vi "ScaleRawData.vi"(4 "Vx,Vy,Vsum as signals or\ntrue X,Y,Z signal (1,default)":bool=TRUE, 5 "error in (no error)":errorcluster, 6 "All DAQ channels":T3, 7 "Scale Option":i32(ring)=2 items=["ScaleButDoNotCalculatePsi", "CalculatePsi, ButDoNotCompensate", "CompensationAllSignalsByCalcuatedPsi", "DoNotScale(ReadRawVoltageSignals)"], 8 "Params in":T8={"TaskIDs"={"DAQ tasks"={"Px taskID"=0, "Py taskID"=0, "Pz taskID"=0, "AOM taskID"=0, "Clock taskID"=0, "AI taskID"=0}, "DVEHandle"=refnum}, "Manual Control"={"Rotation Control"={"Phase"=0.0, "A amp (0-120)"=75.0, "B amp (0-120)"=53.3, "mean freq  [MHz]\ndefault 39.99"=40.0, "freq difference [Hz]"=2.0, "Enable A"=TRUE, "Enable B"=TRUE}, "X piezo\n [nm]"=0.0, "Y peizo\n [nm]"=0.0, "trap height\n [nm]"=5.012658227848101, "AOM0 \nPower"=0.2}, "Piezo Calibr"={"Px2Vx(AO)"=nan, "Py2Vy(AO)"=nan, "Pz2Vz(AO)"=nan, "Min Px"=nan, "Min Py"=nan, "Min Pz"=nan, "Max Px"=nan, "Max Py"=nan, "Max Pz"=nan, "Vx0 (V)"=nan, "Vy0 (V)"=nan, "Vz0 (V)"=nan}, "Instrument Calibr"={"Angular compensation coeffs"=[], "TetherCenter"={"TrapX_AO 0 [nm]"=nan, "TrapY_AO 0 [nm]"=nan, "TrapZ_AO 0 [nm]"=nan}, "XYZsignal baseline"={"Xsignal0"=nan, "Ysignal0"=nan, "Zsignal0"=nan, "Zsig slope"=nan, "Z bead0"=nan}, "S and P to Vs0"={"Vs0/P"=1.0, "Vs0/S"=1.0}, "Psi"=0.0, "ePS:eRL drift correlation"={"Interc P"=nan, "Slope P"=nan, "Interc S"=nan, "Slope S"=nan}, "Current piezo volt AO"={"Vpx_AO [V]"=nan, "Vpy_AO [V]"=nan, "Vpz_AO [V]"=nan}}, "Cylinder Calibr"={"ZStiff"=nan, "Zsens"=nan, "AngStiff"=nan, "XStiff"=nan, "Xsens"=nan, "MaxEllip"=nan, "YStiff"=nan, "Ysens"=nan, "FocalShift"=nan, "Sfz"=nan, "1/Sz"=nan, "Stau"=nan, "Sfx"=nan, "1/Sx"=nan, "1/Sang"=nan, "Sfy"=nan, "1/Sy"=nan, "1/focal"=nan, "ZsignalHeightDependence (1/nm)"=0.0}, "DAQParams"={"Buffer size"=nan, "Scanning rate"=nan, "Average"=nan, "Sampling rate"=nan, "set dt"=nan}, "DAQ channel offsets"={"A0 [V]"=0.0, "D0 [V]"=0.0, "P0  [V]"=0.0, "S0 [V]"=0.0, "L0 [V]"=0.0, "R0 [V]"=0.0, "Vpx0 [V]"=0.0, "Vpy0 [V]"=0.0, "Vpz0 [V]"=0.0, "Vsum0 [V]"=0.0, "Vpx_AO0 [V]"=0.0, "Vpy_AO0 [V]"=0.0, "Vpz_AO0 [V]"=0.0}, "Z bead polynomial coeffs"=[nan, nan, nan, nan], "Skip button ref"=refnum, "z bead lookup table"={"z signal"=[], "z bead"=[]}, "SP->power Matrix"=[], "Ms2p"=[], "Mp2s"=[], "Polynomial coeff V_px,y,z 2 position (nm)"=[]} {"Cylinder Calibr"."ZsignalHeightDependence (1/nm)" format="%.4e"; "Instrument Calibr"."Psi" format="%#_2f"; "Manual Control"."Y peizo\n [nm]" step=100.0 scale=0.0..30000.0; "Manual Control"."AOM0 \nPower" scale=0.0..1.0; "Manual Control"."X piezo\n [nm]" step=100.0 scale=0.0..30000.0; "Manual Control"."Rotation Control"."mean freq  [MHz]\ndefault 39.99" min=0.0 step=0.01; "Manual Control"."Rotation Control"."B amp (0-120)" min=0.0 max=120.0 step=0.1 format="%.1f"; "Manual Control"."Rotation Control"."A amp (0-120)" min=0.0 max=120.0 step=0.1 format="%.1f"; "Manual Control"."Rotation Control"."Phase" scale=0.0..360.0; "Manual Control"."trap height\n [nm]" scale=1000.0..7500.0; "TaskIDs"."DAQ tasks"."Px taskID" format="%x"; "TaskIDs"."DAQ tasks"."Py taskID" format="%x"; "TaskIDs"."DAQ tasks"."Pz taskID" format="%x"; "TaskIDs"."DAQ tasks"."AOM taskID" format="%x"; "TaskIDs"."DAQ tasks"."Clock taskID" format="%x"; "TaskIDs"."DAQ tasks"."AI taskID" format="%x"}) -> (0 "error out":errorcluster, 1 "Scaled data":T7, 2 "All DAQ channels out":T3, 3 "Params out":T8={"TaskIDs"={"DAQ tasks"={"Px taskID"=0, "Py taskID"=0, "Pz taskID"=0, "AOM taskID"=0, "Clock taskID"=0, "AI taskID"=0}, "DVEHandle"=refnum}, "Manual Control"={"Rotation Control"={"Phase"=0.0, "A amp (0-120)"=75.0, "B amp (0-120)"=53.3, "mean freq  [MHz]\ndefault 39.99"=40.0, "freq difference [Hz]"=2.0, "Enable A"=TRUE, "Enable B"=TRUE}, "X piezo\n [nm]"=0.0, "Y peizo\n [nm]"=0.0, "trap height\n [nm]"=5.012658227848101, "AOM0 \nPower"=0.2}, "Piezo Calibr"={"Px2Vx(AO)"=nan, "Py2Vy(AO)"=nan, "Pz2Vz(AO)"=nan, "Min Px"=nan, "Min Py"=nan, "Min Pz"=nan, "Max Px"=nan, "Max Py"=nan, "Max Pz"=nan, "Vx0 (V)"=nan, "Vy0 (V)"=nan, "Vz0 (V)"=nan}, "Instrument Calibr"={"Angular compensation coeffs"=[], "TetherCenter"={"TrapX_AO 0 [nm]"=nan, "TrapY_AO 0 [nm]"=nan, "TrapZ_AO 0 [nm]"=nan}, "XYZsignal baseline"={"Xsignal0"=nan, "Ysignal0"=nan, "Zsignal0"=nan, "Zsig slope"=nan, "Z bead0"=nan}, "S and P to Vs0"={"Vs0/P"=1.0, "Vs0/S"=1.0}, "Psi"=0.0, "ePS:eRL drift correlation"={"Interc P"=nan, "Slope P"=nan, "Interc S"=nan, "Slope S"=nan}, "Current piezo volt AO"={"Vpx_AO [V]"=nan, "Vpy_AO [V]"=nan, "Vpz_AO [V]"=nan}}, "Cylinder Calibr"={"ZStiff"=nan, "Zsens"=nan, "AngStiff"=nan, "XStiff"=nan, "Xsens"=nan, "MaxEllip"=nan, "YStiff"=nan, "Ysens"=nan, "FocalShift"=nan, "Sfz"=nan, "1/Sz"=nan, "Stau"=nan, "Sfx"=nan, "1/Sx"=nan, "1/Sang"=nan, "Sfy"=nan, "1/Sy"=nan, "1/focal"=nan, "ZsignalHeightDependence (1/nm)"=0.0}, "DAQParams"={"Buffer size"=nan, "Scanning rate"=nan, "Average"=nan, "Sampling rate"=nan, "set dt"=nan}, "DAQ channel offsets"={"A0 [V]"=0.0, "D0 [V]"=0.0, "P0  [V]"=0.0, "S0 [V]"=0.0, "L0 [V]"=0.0, "R0 [V]"=0.0, "Vpx0 [V]"=0.0, "Vpy0 [V]"=0.0, "Vpz0 [V]"=0.0, "Vsum0 [V]"=0.0, "Vpx_AO0 [V]"=0.0, "Vpy_AO0 [V]"=0.0, "Vpz_AO0 [V]"=0.0}, "Z bead polynomial coeffs"=[nan, nan, nan, nan], "Skip button ref"=refnum, "z bead lookup table"={"z signal"=[], "z bead"=[]}, "SP->power Matrix"=[], "Ms2p"=[], "Mp2s"=[], "Polynomial coeff V_px,y,z 2 position (nm)"=[]} {"Cylinder Calibr"."ZsignalHeightDependence (1/nm)" format="%.4e"; "Instrument Calibr"."Psi" format="%#_2f"; "Manual Control"."Y peizo\n [nm]" step=100.0 scale=0.0..30000.0; "Manual Control"."AOM0 \nPower" scale=0.0..1.0; "Manual Control"."X piezo\n [nm]" step=100.0 scale=0.0..30000.0; "Manual Control"."Rotation Control"."mean freq  [MHz]\ndefault 39.99" min=0.0 step=0.01; "Manual Control"."Rotation Control"."B amp (0-120)" min=0.0 max=120.0 step=0.1 format="%.1f"; "Manual Control"."Rotation Control"."A amp (0-120)" min=0.0 max=120.0 step=0.1 format="%.1f"; "Manual Control"."Rotation Control"."Phase" scale=0.0..360.0; "Manual Control"."trap height\n [nm]" scale=1000.0..7500.0; "TaskIDs"."DAQ tasks"."Px taskID" format="%x"; "TaskIDs"."DAQ tasks"."Py taskID" format="%x"; "TaskIDs"."DAQ tasks"."Pz taskID" format="%x"; "TaskIDs"."DAQ tasks"."AOM taskID" format="%x"; "TaskIDs"."DAQ tasks"."Clock taskID" format="%x"; "TaskIDs"."DAQ tasks"."AI taskID" format="%x"})   [LabVIEW 2020, in "SignalConverson.lvlib"]
uses:
  SignalConverson.lvlib
  Initialization/Param.ctl
  Initialization/ManualCtrl.ctl
  Initialization/DVESetting.ctl
  Initialization/CylinderCalibrNew.ctl
  DAQChannelOffsets.ctl
  <vilib>/Analysis/Matrix/Datatypes/RealMatrix.ctl
  DAQChannelRawData.ctl
  ScaledData.ctl
  Measrured TrapXYZ.ctl
  Data Before Angle Compensation.ctl
  Angle compensated data.ctl
  XYZ Signals.ctl
  Set TrapXYZ.ctl
  <vilib>/Analysis/baseanly.llb/A x Vector.vi
  <vilib>/Analysis/polynomials.llb/Scalar Polynomial Evaluation (DBL).vi
  <vilib>/Analysis/NI_AALBase.lvlib
  <vilib>/Analysis/NI_AALPro.lvlib
  Initialization/Initialization.lvlib
  <vilib>/Analysis/Matrix/NI_Matrix.lvlib
panel:
  out "Data before TCT":T1
  out "set TrapXYZ":T2
  out "Measured Piezo Position":T4
  out "X,Y,Z signal":T5
  out "Data after TCT":T6
  out "Data Before TCT":T1
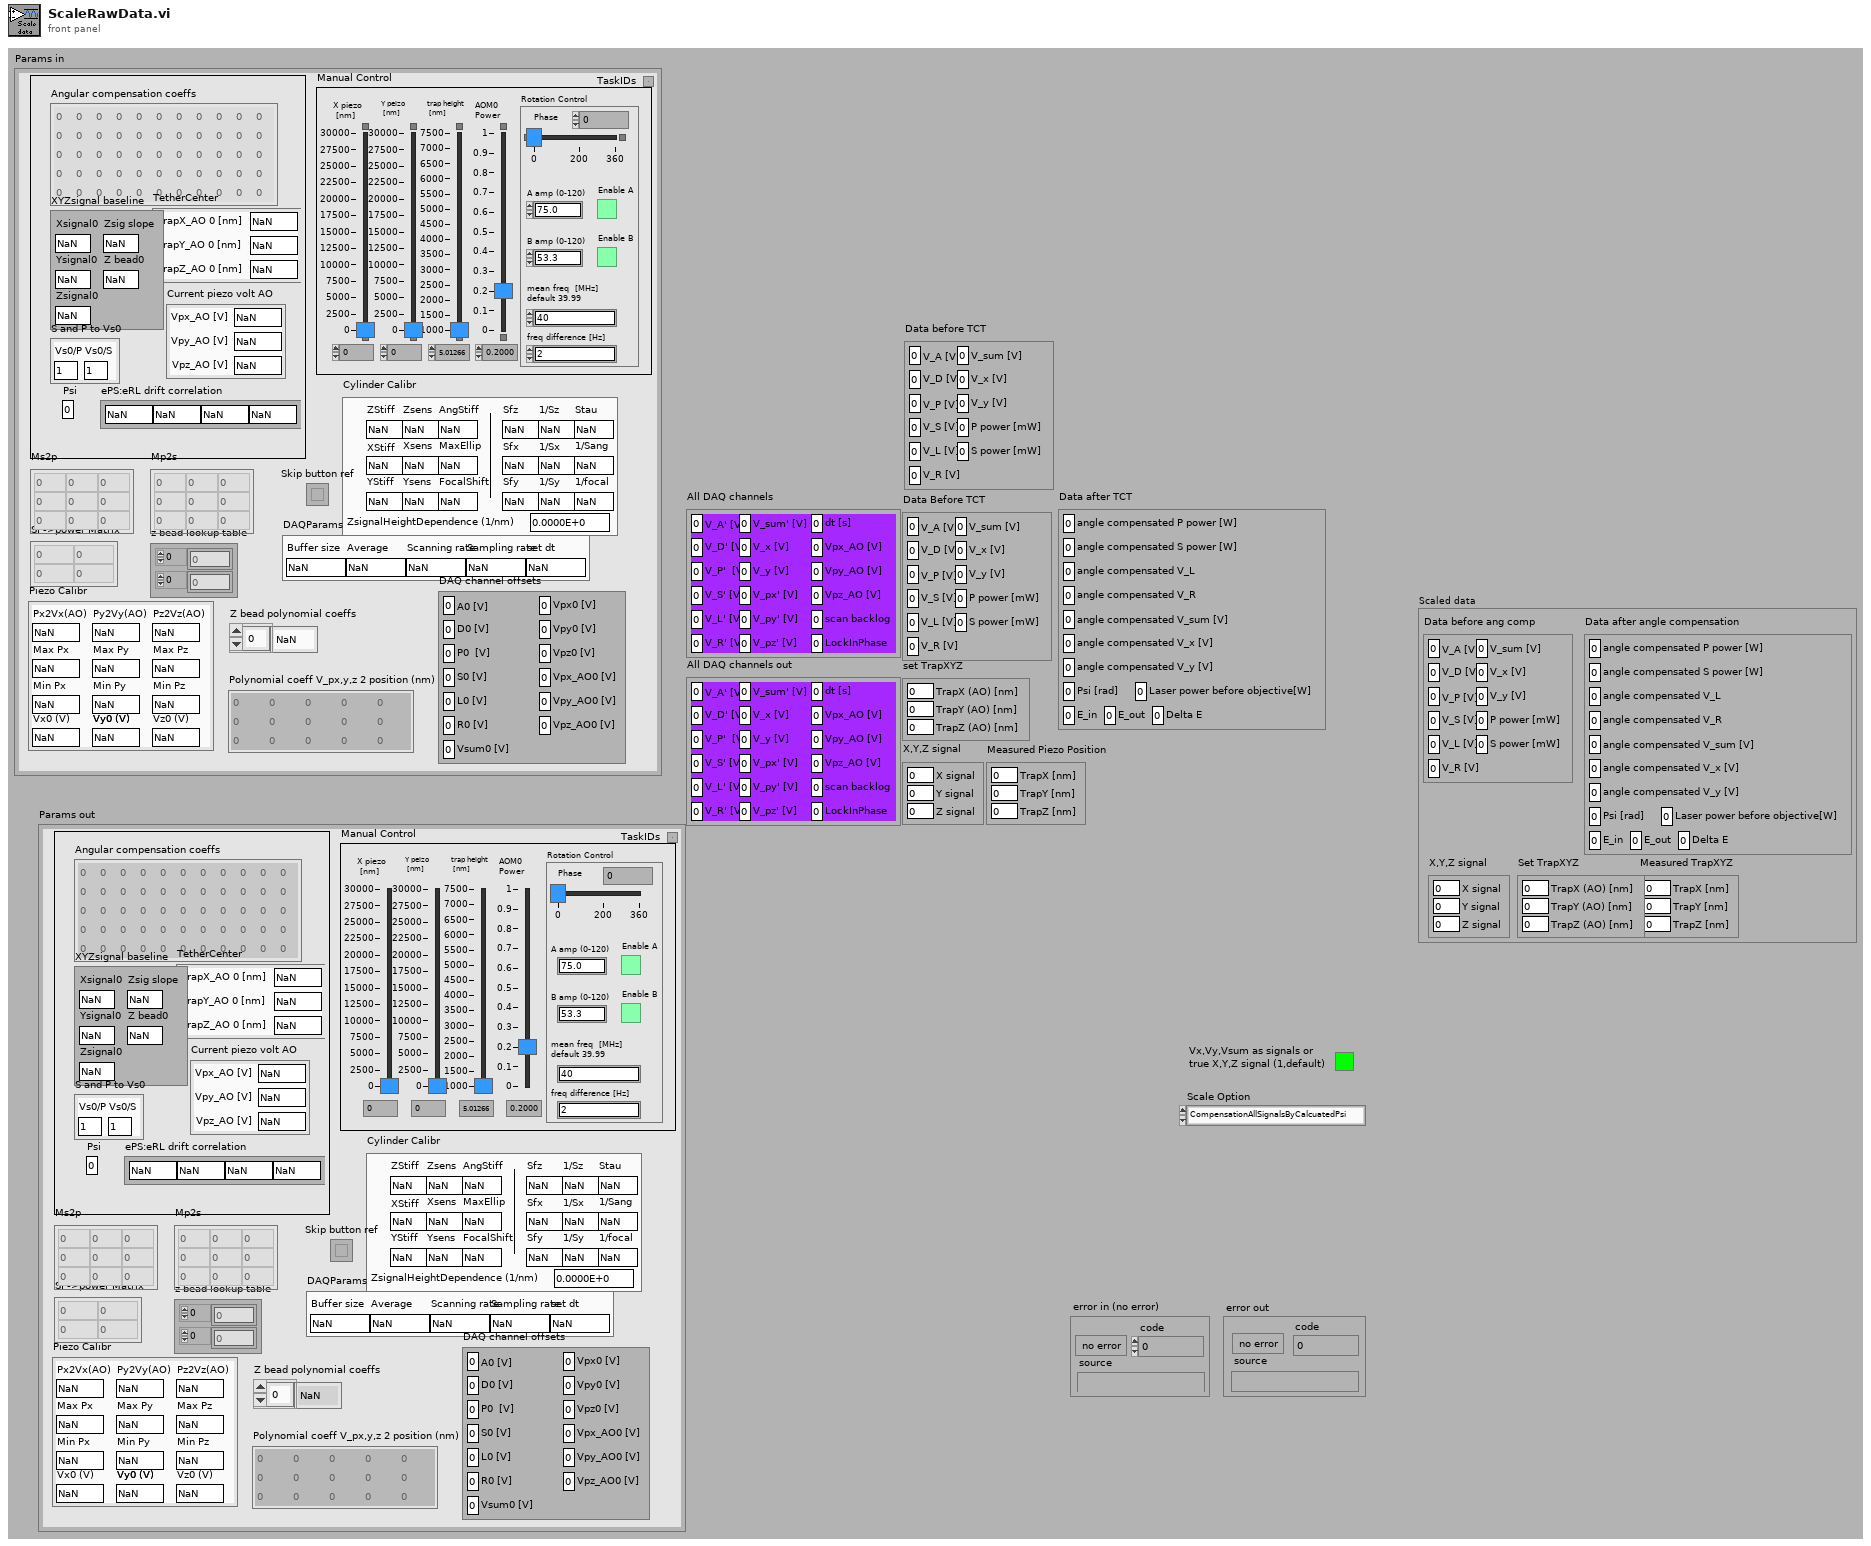
[diagram p1: front panel]
types:
  T1 = typedef "SignalConverson.lvlib/Data Before Angle Compensation.ctl" = cluster{"V_A [V]":dbl, "V_D [V]":dbl, "V_P [V]":dbl, "V_S [V]":dbl, "V_L [V]":dbl, "V_R [V]":dbl, "V_sum [V]":dbl, "V_x [V]":dbl, "V_y [V]":dbl, "P power [mW]":dbl, "S power [mW]":dbl}
  T2 = typedef "SignalConverson.lvlib/Set TrapXYZ.ctl" = cluster{"TrapX (AO) [nm]":dbl, "TrapY (AO) [nm]":dbl, "TrapZ (AO) [nm]":dbl}
  T3 = typedef "SignalConverson.lvlib/DAQChannelRawData.ctl" = cluster{"V_A' [V]":dbl, "V_D' [V]":dbl, "V_P'  [V]":dbl, "V_S' [V]":dbl, "V_L' [V]":dbl, "V_R' [V]":dbl, "V_sum' [V]":dbl, "V_x [V]":dbl, "V_y [V]":dbl, "V_px' [V]":dbl, "V_py' [V]":dbl, "V_pz' [V]":dbl, "dt [s]":dbl, "Vpx_AO [V]":dbl, "Vpy_AO [V]":dbl, "Vpz_AO [V]":dbl, "scan backlog":u32, "LockInPhase":dbl}
  T4 = typedef "SignalConverson.lvlib/Measrured TrapXYZ.ctl" = cluster{"TrapX [nm]":dbl, "TrapY [nm]":dbl, "TrapZ [nm]":dbl}
  T5 = typedef "SignalConverson.lvlib/XYZ Signals.ctl" = cluster{"X signal":dbl, "Y signal":dbl, "Z signal":dbl}
  T6 = typedef "SignalConverson.lvlib/Angle compensated data.ctl" = cluster{"angle compensated P power [W]":dbl, "angle compensated S power [W]":dbl, "angle compensated V_L":dbl, "angle compensated V_R":dbl, "angle compensated V_sum [V]":dbl, "angle compensated V_x [V]":dbl, "angle compensated V_y [V]":dbl, "Psi [rad]":dbl, "Laser power before objective[W]":dbl, "E_in":dbl, "E_out":dbl, "Delta E":dbl}
  T7 = typedef "SignalConverson.lvlib/ScaledData.ctl" = cluster{"Measured TrapXYZ":T4, "Data before ang comp":T1, "Data after angle compensation":T6, "X,Y,Z signal":T5, "Set TrapXYZ":T2}
  T8 = typedef "Initialization.lvlib/Param.ctl" = cluster{"TaskIDs":cluster{"DAQ tasks":cluster{"Px taskID":u32, "Py taskID":u32, "Pz taskID":u32, "AOM taskID":u32, "Clock taskID":u32, "AI taskID":u32}, "DVEHandle":refnum<file>}, "Manual Control":T9, "Piezo Calibr":cluster{"Px2Vx(AO)":dbl, "Py2Vy(AO)":dbl, "Pz2Vz(AO)":dbl, "Min Px":dbl, "Min Py":dbl, "Min Pz":dbl, "Max Px":dbl, "Max Py":dbl, "Max Pz":dbl, "Vx0 (V)":dbl, "Vy0 (V)":dbl, "Vz0 (V)":dbl}, "Instrument Calibr":cluster{"Angular compensation coeffs":dbl[][], "TetherCenter":cluster{"TrapX_AO 0 [nm]":dbl, "TrapY_AO 0 [nm]":dbl, "TrapZ_AO 0 [nm]":dbl}, "XYZsignal baseline":cluster{"Xsignal0":dbl, "Ysignal0":dbl, "Zsignal0":dbl, "Zsig slope":dbl, "Z bead0":dbl}, "S and P to Vs0":cluster{"Vs0/P":dbl, "Vs0/S":dbl}, "Psi":dbl, "ePS:eRL drift correlation":cluster{"Interc P":dbl, "Slope P":dbl, "Interc S":dbl, "Slope S":dbl}, "Current piezo volt AO":cluster{"Vpx_AO [V]":dbl, "Vpy_AO [V]":dbl, "Vpz_AO [V]":dbl}}, "Cylinder Calibr":T11, "DAQParams":cluster{"Buffer size":dbl, "Scanning rate":dbl, "Average":dbl, "Sampling rate":dbl, "set dt":dbl}, "DAQ channel offsets":T12, "Z bead polynomial coeffs":dbl[], "Skip button ref":refnum<vi>, "z bead lookup table":cluster{"z signal":dbl[], "z bead":dbl[]}, "SP->power Matrix":T13, "Ms2p":T13, "Mp2s":T13, "Polynomial coeff V_px,y,z 2 position (nm)":dbl[][]}
  T9 = typedef "Initialization.lvlib/ManualCtrl.ctl" = cluster{"Rotation Control":T10, "X piezo\n [nm]":dbl, "Y peizo\n [nm]":dbl, "trap height\n [nm]":dbl, "AOM0 \nPower":dbl}
  T10 = typedef "Initialization.lvlib/DVESetting.ctl" = cluster{"Phase":dbl, "A amp (0-120)":dbl, "B amp (0-120)":dbl, "mean freq  [MHz]\ndefault 39.99":dbl, "freq difference [Hz]":dbl, "Enable A":bool, "Enable B":bool}
  T11 = typedef "Initialization.lvlib/CylinderCalibrNew.ctl" = cluster{"ZStiff":dbl, "Zsens":dbl, "AngStiff":dbl, "XStiff":dbl, "Xsens":dbl, "MaxEllip":dbl, "YStiff":dbl, "Ysens":dbl, "FocalShift":dbl, "Sfz":dbl, "1/Sz":dbl, "Stau":dbl, "Sfx":dbl, "1/Sx":dbl, "1/Sang":dbl, "Sfy":dbl, "1/Sy":dbl, "1/focal":dbl, "ZsignalHeightDependence (1/nm)":dbl}
  T12 = typedef "SignalConverson.lvlib/DAQChannelOffsets.ctl" = cluster{"A0 [V]":dbl, "D0 [V]":dbl, "P0  [V]":dbl, "S0 [V]":dbl, "L0 [V]":dbl, "R0 [V]":dbl, "Vpx0 [V]":dbl, "Vpy0 [V]":dbl, "Vpz0 [V]":dbl, "Vsum0 [V]":dbl, "Vpx_AO0 [V]":dbl, "Vpy_AO0 [V]":dbl, "Vpz_AO0 [V]":dbl}
  T13 = typedef "NI_Matrix.lvlib/RealMatrix.ctl" = dbl[][]
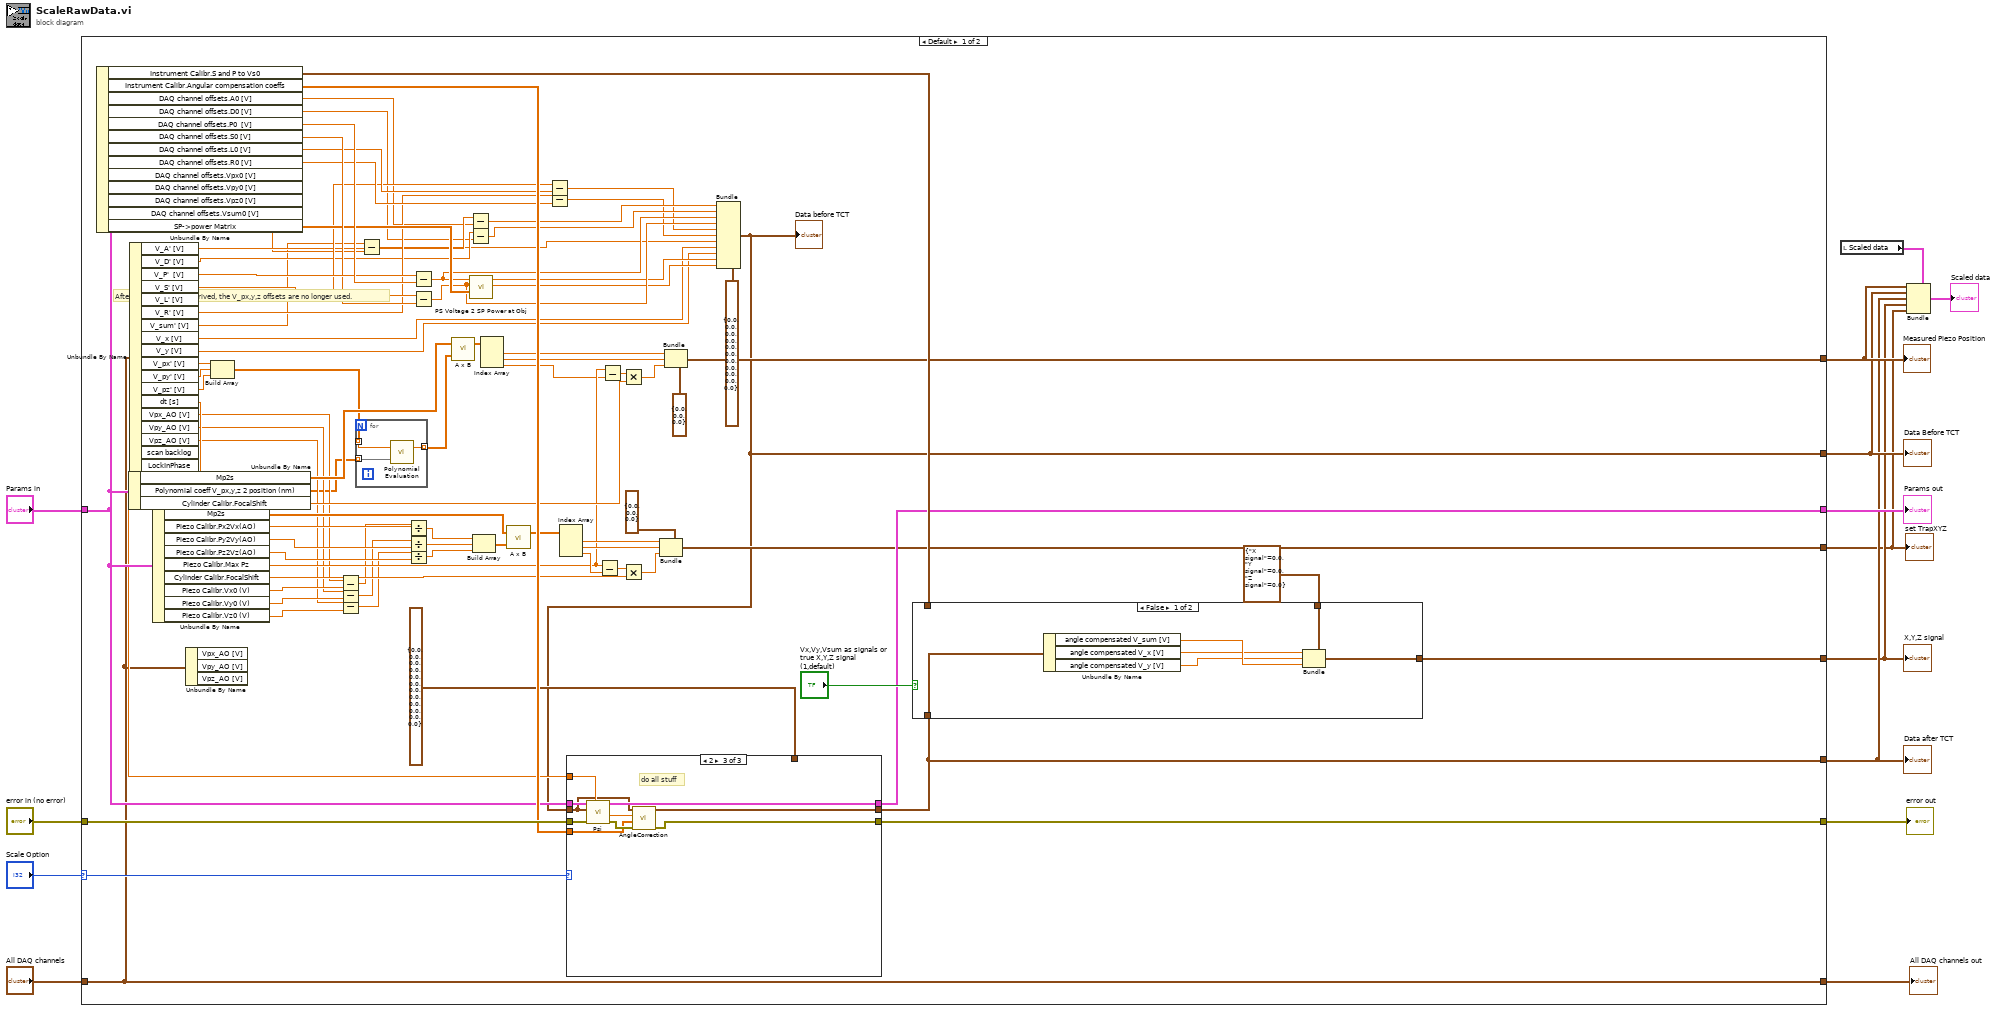
[diagram p0: block diagram]
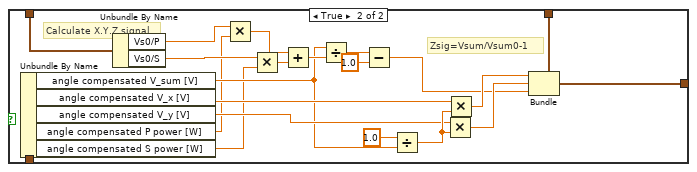
[diagram p2: hidden frame]
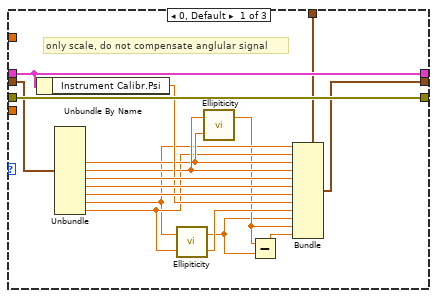
[diagram p3: hidden frame]
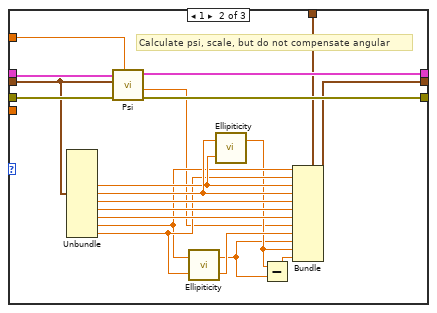
[diagram p4: hidden frame]
diagram:
  n1 = case shown="Default" "Scale Option" {
    selector: "Scale Option" -> [w96 _]
    tunnel: "All DAQ channels" -> [w50 w177]
    tunnel: "Params in" -> [w84 w178]
    tunnel: "error in (no error)" -> [w99 w179]
    tunnel: [w97 w179] -> w2
    tunnel: [w93 w178] -> w13
    tunnel: [w56 _] -> w4
    tunnel: [w55 _] -> w5
    tunnel: [w40 _] -> w6
    tunnel: [w51 _] -> w7
    tunnel: [w50 w177] -> w9
    tunnel: [w41 _] -> w3
    frame Default {
      # "After the new PI piezo arrived, the V_px,y,z offsets are no longer used."
      n2 = Unbundle By Name(w84) -> ("Instrument Calibr.S and P to Vs0"=w95:cluster{"Vs0/P":dbl, "Vs0/S":dbl}, "Instrument Calibr.Angular compensation coeffs"=w98:dbl[][], "DAQ channel offsets.A0 [V]"=w69:dbl, "DAQ channel offsets.D0 [V]"=w68:dbl, "DAQ channel offsets.P0  [V]"=w92:dbl, "DAQ channel offsets.S0 [V]"=w89:dbl, "DAQ channel offsets.L0 [V]"=w82:dbl, "DAQ channel offsets.R0 [V]"=w83:dbl, "DAQ channel offsets.Vsum0 [V]"=w38:dbl, "SP->power Matrix"=w88:T13)  [unwired: 3 out]
      n3 = Unbundle By Name(w84) -> ("Mp2s"=w85:T13, "Polynomial coeff V_px,y,z 2 position (nm)"=w22:dbl[][], "Cylinder Calibr.FocalShift"=w86:dbl)
      n4 = Unbundle By Name(w50) -> ("V_A' [V]"=w71:dbl, "V_D' [V]"=w70:dbl, "V_P'  [V]"=w91:dbl, "V_S' [V]"=w90:dbl, "V_L' [V]"=w81:dbl, "V_R' [V]"=w80:dbl, "V_sum' [V]"=w37:dbl, "V_x [V]"=w61:dbl, "V_y [V]"=w60:dbl, "V_px' [V]"=w19:dbl, "V_py' [V]"=w18:dbl, "V_pz' [V]"=w17:dbl, "dt [s]"=w59:dbl, "Vpx_AO [V]"=w28:dbl, "Vpy_AO [V]"=w27:dbl, "Vpz_AO [V]"=w26:dbl)  [unwired: 2 out]
      n5 = Unbundle By Name(w84) -> ("Mp2s"=w73:T13, "Piezo Calibr.Px2Vx(AO)"=w79:dbl, "Piezo Calibr.Py2Vy(AO)"=w78:dbl, "Piezo Calibr.Pz2Vz(AO)"=w77:dbl, "Piezo Calibr.Max Pz"=w35:dbl, "Cylinder Calibr.FocalShift"=w46:dbl, "Piezo Calibr.Vx0 (V)"=w31:dbl, "Piezo Calibr.Vy0 (V)"=w30:dbl, "Piezo Calibr.Vz0 (V)"=w29:dbl)
      n6 = Unbundle By Name(w50) -> ()  [unwired: 3 out]
      n7 = Build Array(w19, w18, w17) -> (w21:dbl[])
      n8 = Subtract(x=w28, y=w31) -> (x-y=w25:dbl)
      n9 = Subtract(x=w27, y=w30) -> (x-y=w24:dbl)
      n10 = Subtract(x=w26, y=w29) -> (x-y=w23:dbl)
      n11 = for {
        tunnel: w22 -> [w101] mode=indexing
        tunnel: w21 -> [w102] mode=indexing
        tunnel: [w100] -> w20 mode=indexing
        n12 = call-poly <vilib>:"Polynomial Evaluation.vi"("P(x)"=w101, "a"=w102) -> ("P(a)"=w100:dbl)  [unwired: 1 out]
      }
      n13 = Subtract(x=w37, y=w38) -> (x-y=w36:dbl)
      n14 = Divide(x=w25, y=w79) -> (x/y=w75:dbl)
      n15 = Divide(x=w24, y=w78) -> (x/y=w76:dbl)
      n16 = Divide(x=w23, y=w77) -> (x/y=w49:dbl)
      n17 = Subtract(x=w91, y=w92) -> (x-y=w65:dbl)
      n18 = Subtract(x=w90, y=w89) -> (x-y=w64:dbl)
      n19 = call-poly <vilib>:"A x B.vi"("Vector"=w20, "A"=w85) -> ("A x Vector"=w87:dbl[])  [unwired: 1 out]
      n20 = Subtract(x=w71, y=w69) -> (x-y=w67:dbl)
      n21 = Subtract(x=w70, y=w68) -> (x-y=w66:dbl)
      n22 = call "PS Voltage 2 SP Power at Obj.vi"("SP -> Power Matrix"=w88, "Volts S"=w64, "Volts P"=w65) -> ("Power S"=w62:dbl, "Power P"=w63:dbl)  [unwired: 3 in]
      n23 = Build Array(w75, w76, w49) -> (w74:dbl[])
      n24 = Index Array(array=w87) -> (element #1=w53:dbl, element #2=w52:dbl, element #3=w34:dbl)  [unwired: 3 in]
      n25 = call-poly <vilib>:"A x B.vi"("Vector"=w74, "A"=w73) -> ("A x Vector"=w72:dbl[])  [unwired: 1 out]
      n26 = Subtract(x=w81, y=w82) -> (x-y=w16:dbl)
      n27 = Subtract(x=w80, y=w83) -> (x-y=w15:dbl)
      n28 = Index Array(array=w72) -> (element #1=w45:dbl, element #2=w44:dbl, element #3=w48:dbl)  [unwired: 3 in]
      n29 = Subtract(x=w35, y=w48) -> (x-y=w47:dbl)
      n30 = Subtract(x=w35, y=w34) -> (x-y=w33:dbl)
      n31 = Multiply(x=w47, y=w46) -> (x*y=w43:dbl)
      n32 = Multiply(x=w33, y=w86) -> (x*y=w32:dbl)
      n33 = Bundle(cluster=T2 {"TrapX (AO) [nm]"=0.0, "TrapY (AO) [nm]"=0.0, "TrapZ (AO) [nm]"=0.0} ("set TrapXYZ"), "TrapX (AO) [nm]"=w45, "TrapY (AO) [nm]"=w44, "TrapZ (AO) [nm]"=w43) -> (w41:T2)
      n34 = Bundle(cluster=T4 {"TrapX [nm]"=0.0, "TrapY [nm]"=0.0, "TrapZ [nm]"=0.0} ("Measured Piezo Position"), "TrapX [nm]"=w53, "TrapY [nm]"=w52, "TrapZ [nm]"=w32) -> (w51:T4)
      n35 = Bundle(cluster=T1 {"V_A [V]"=0.0, "V_D [V]"=0.0, "V_P [V]"=0.0, "V_S [V]"=0.0, "V_L [V]"=0.0, "V_R [V]"=0.0, "V_sum [V]"=0.0, "V_x [V]"=0.0, "V_y [V]"=0.0, "P power [mW]"=0.0, "S power [mW]"=0.0} ("Data before TCT"), "V_A [V]"=w67, "V_D [V]"=w66, "V_P [V]"=w65, "V_S [V]"=w64, "V_L [V]"=w16, "V_R [V]"=w15, "V_sum [V]"=w36, "V_x [V]"=w61, "V_y [V]"=w60, "P power [mW]"=w63, "S power [mW]"=w62) -> (w40:T1)
      "Data before TCT" <- w40
      n36 = case shown="2" w96 {
        tunnel: w99 -> [w146 w165 w175]
        tunnel: [w138 w148 w168] -> w55
        tunnel: [w146 w166 w174] -> w97
        tunnel: w98 -> [_ _ w173]
        tunnel: w84 -> [w145 w164 w172]
        tunnel: [w145 w163 w171] -> w93
        tunnel: w40 -> [w144 w150 w167]
        tunnel: w59 -> [_ w162 w169]
        tunnel: T6 {"angle compensated P power [W]"=0.0, "angle compensated S power [W]"=0.0, "angle compensated V_L"=0.0, "angle compensated V_R"=0.0, "angle compensated V_sum [V]"=0.0, "angle compensated V_x [V]"=0.0, "angle compensated V_y [V]"=0.0, "Psi [rad]"=0.0, "Laser power before objective[W]"=0.0, "E_in"=0.0, "E_out"=0.0, "Delta E"=0.0} ("Data after TCT") -> [w143 w149 _]
        frame 0, Default {
          # "only scale, do not compensate anglular signal"
          n37 = Unbundle By Name(w145) -> ("Instrument Calibr.Psi"=w139:dbl)
          n38 = Unbundle(w144) -> ("V_L [V]"=w136:dbl, "V_R [V]"=w137:dbl, "V_sum [V]"=w142:dbl, "V_x [V]"=w141:dbl, "V_y [V]"=w140:dbl, "P power [mW]"=w134:dbl, "S power [mW]"=w135:dbl)  [unwired: 4 out]
          n39 = call "Ellipiticity.vi"("S or L"=w135, "P or R"=w134) -> ("P+S"=w133:dbl, "(P-S)/(P+S)"=w131:dbl)
          n40 = call "Ellipiticity.vi"("S or L"=w136, "P or R"=w137) -> ("(P-S)/(P+S)"=w132:dbl)  [unwired: 1 out]
          n41 = Subtract(x=w132, y=w131) -> (x-y=w130:dbl)
          n42 = Bundle(cluster=w143, "angle compensated P power [W]"=w134, "angle compensated S power [W]"=w135, "angle compensated V_L"=w136, "angle compensated V_R"=w137, "angle compensated V_sum [V]"=w142, "angle compensated V_x [V]"=w141, "angle compensated V_y [V]"=w140, "Psi [rad]"=w139, "Laser power before objective[W]"=w133, "E_in"=w131, "E_out"=w132, "Delta E"=w130) -> (w138:T6)
        }
        frame 1 {
          # "Calculate psi, scale, but do not compensate angular"
          n43 = Unbundle(w150) -> ("V_L [V]"=w157:dbl, "V_R [V]"=w158:dbl, "V_sum [V]"=w161:dbl, "V_x [V]"=w160:dbl, "V_y [V]"=w159:dbl, "P power [mW]"=w155:dbl, "S power [mW]"=w156:dbl)  [unwired: 4 out]
          n44 = call "Psi.vi"("dt [s]"=w162, "error in (no error)"=w165, "Data before TCT"=w150, "Params in"=w164) -> ("error out"=w166:errorcluster, "Psi"=w147:dbl, "Params out"=w163:T8)  [unwired: 2 in]
          n45 = call "Ellipiticity.vi"("S or L"=w156, "P or R"=w155) -> ("P+S"=w154:dbl, "(P-S)/(P+S)"=w152:dbl)
          n46 = call "Ellipiticity.vi"("S or L"=w157, "P or R"=w158) -> ("(P-S)/(P+S)"=w153:dbl)  [unwired: 1 out]
          n47 = Subtract(x=w153, y=w152) -> (x-y=w151:dbl)
          n48 = Bundle(cluster=w149, "angle compensated P power [W]"=w155, "angle compensated S power [W]"=w156, "angle compensated V_L"=w157, "angle compensated V_R"=w158, "angle compensated V_sum [V]"=w161, "angle compensated V_x [V]"=w160, "angle compensated V_y [V]"=w159, "Psi [rad]"=w147, "Laser power before objective[W]"=w154, "E_in"=w152, "E_out"=w153, "Delta E"=w151) -> (w148:T6)
        }
        frame 2 {
          # "do all stuff"
          n49 = call "Psi.vi"("dt [s]"=w169, "error in (no error)"=w175, "Data before TCT"=w167, "Params in"=w172) -> ("error out"=w176:errorcluster, "Psi"=w170:dbl, "Params out"=w171:T8)  [unwired: 2 in]
          n50 = call "AngleCorrection.vi"("error in (no error)"=w176, "TQGT"=w173, "Psi"=w170, "Data Before TCT"=w167) -> ("error out"=w174:errorcluster, "Data after TCT"=w168:T6)  [unwired: 2 in]
        }
      }
      n51 = case shown="False" "Vx,Vy,Vsum as signals or\ntrue X,Y,Z signal (1,default)" {
        tunnel: w95 -> [_ w122]
        tunnel: [w107 w111] -> w56
        tunnel: w55 -> [w106 w120]
        tunnel: T5 {"X signal"=0.0, "Y signal"=0.0, "Z signal"=0.0} ("X,Y,Z signal") -> [w108 w110]
        frame False {
          n52 = Unbundle By Name(w106) -> ("angle compensated V_sum [V]"=w105:dbl, "angle compensated V_x [V]"=w104:dbl, "angle compensated V_y [V]"=w103:dbl)
          n53 = Bundle(cluster=w108, "X signal"=w104, "Y signal"=w103, "Z signal"=w105) -> (w107:T5)
        }
        frame True {
          # "Zsig=Vsum/Vsum0-1"
          # "Calculate X.Y.Z signal"
          n54 = Unbundle By Name(w120) -> ("angle compensated V_sum [V]"=w117:dbl, "angle compensated V_x [V]"=w119:dbl, "angle compensated V_y [V]"=w118:dbl, "angle compensated P power [W]"=w116:dbl, "angle compensated S power [W]"=w115:dbl)
          n55 = Unbundle By Name(w122) -> ("Vs0/P"=w125:dbl, "Vs0/S"=w126:dbl)
          n56 = Multiply(x=w125, y=w116) -> (x*y=w128:dbl)
          n57 = Multiply(x=w126, y=w115) -> (x*y=w127:dbl)
          n58 = Add(x=w128, y=w127) -> (x+y=w129:dbl)
          n59 = Divide(x=w117, y=w129) -> (x/y=w109:dbl)
          n60 = Subtract(x=w109, y=1.0 ("x")) -> (x-y=w112:dbl)
          n61 = Divide(x=1.0, y=w117) -> (x/y=w124:dbl)
          n62 = Multiply(x=w118, y=w124) -> (x*y=w113:dbl)
          n63 = Multiply(x=w119, y=w124) -> (x*y=w114:dbl)
          n64 = Bundle(cluster=w110, "X signal"=w114, "Y signal"=w113, "Z signal"=w112) -> (w111:T5)
        }
      }
    }
    frame 3 {
    }
  }
  "Params out" <- w13
  "X,Y,Z signal" <- w4
  "Data after TCT" <- w5
  "Data Before TCT" <- w6
  "Measured Piezo Position" <- w7
  "All DAQ channels out" <- w9
  "set TrapXYZ" <- w3
  "error out" <- w2
  n65 = local read "Scaled data"() -> (w8:T7)
  n66 = Bundle(cluster=w8, "Measured TrapXYZ"=w7, "Data before ang comp"=w6, "Data after angle compensation"=w5, "X,Y,Z signal"=w4, "Set TrapXYZ"=w3) -> (→"Scaled data":T7)
